vi "HW3_2017_BEEP.vi"() -> ()   [LabVIEW 2017]
panel:
  in  "OK Button 2":bool
  in  "Path":path
  in  "min":dbl
  in  "hour":dbl
  in  "OK Button":bool
  out "Boolean":bool
  in  "SET ALARM":bool
  out "ALARMING TIME":string
  out "DATE":string
  in  "reinstate":bool
  in  "sec":dbl
  in  "min":dbl
  in  "hour":dbl
  in  "reset":bool
  out "sec":dbl(knob) scale=0.0..60.0
  out "min":dbl(knob) scale=0.0..60.0
  out "hour":dbl(knob) scale=0.0..12.0
  in  "stop":bool
  out "new picture":picture
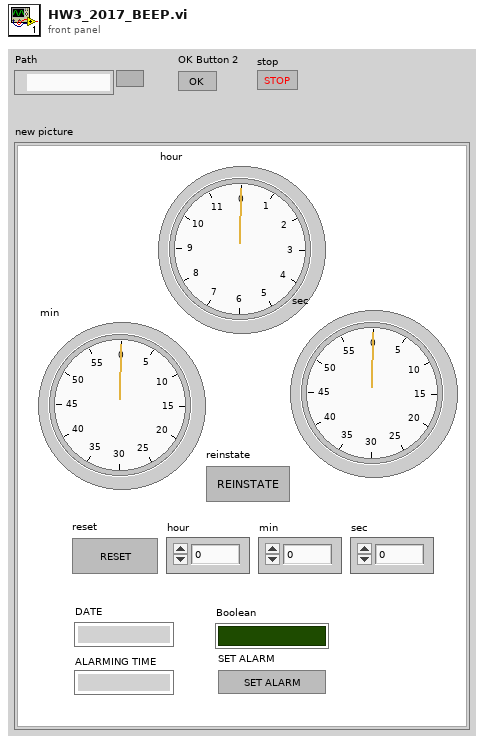
[diagram p1: front panel]
types:
  T1 = typedef "LVDateTimeRec.ctl" = cluster{"fractional second":dbl, "second":i32, "minute":i32, "hour":i32, "day of month":i32, "month":i32, "year":i32, "day of week":i32, "day of year":i32, "DST":i32}
  T2 = typedef "imagedata.ctl" = cluster{"image type":i32, "image depth":i32, "image":u8[], "mask":u8[], "colors":u32[], "Rectangle":cluster{"left":i16, "top":i16, "right":i16, "bottom":i16}}
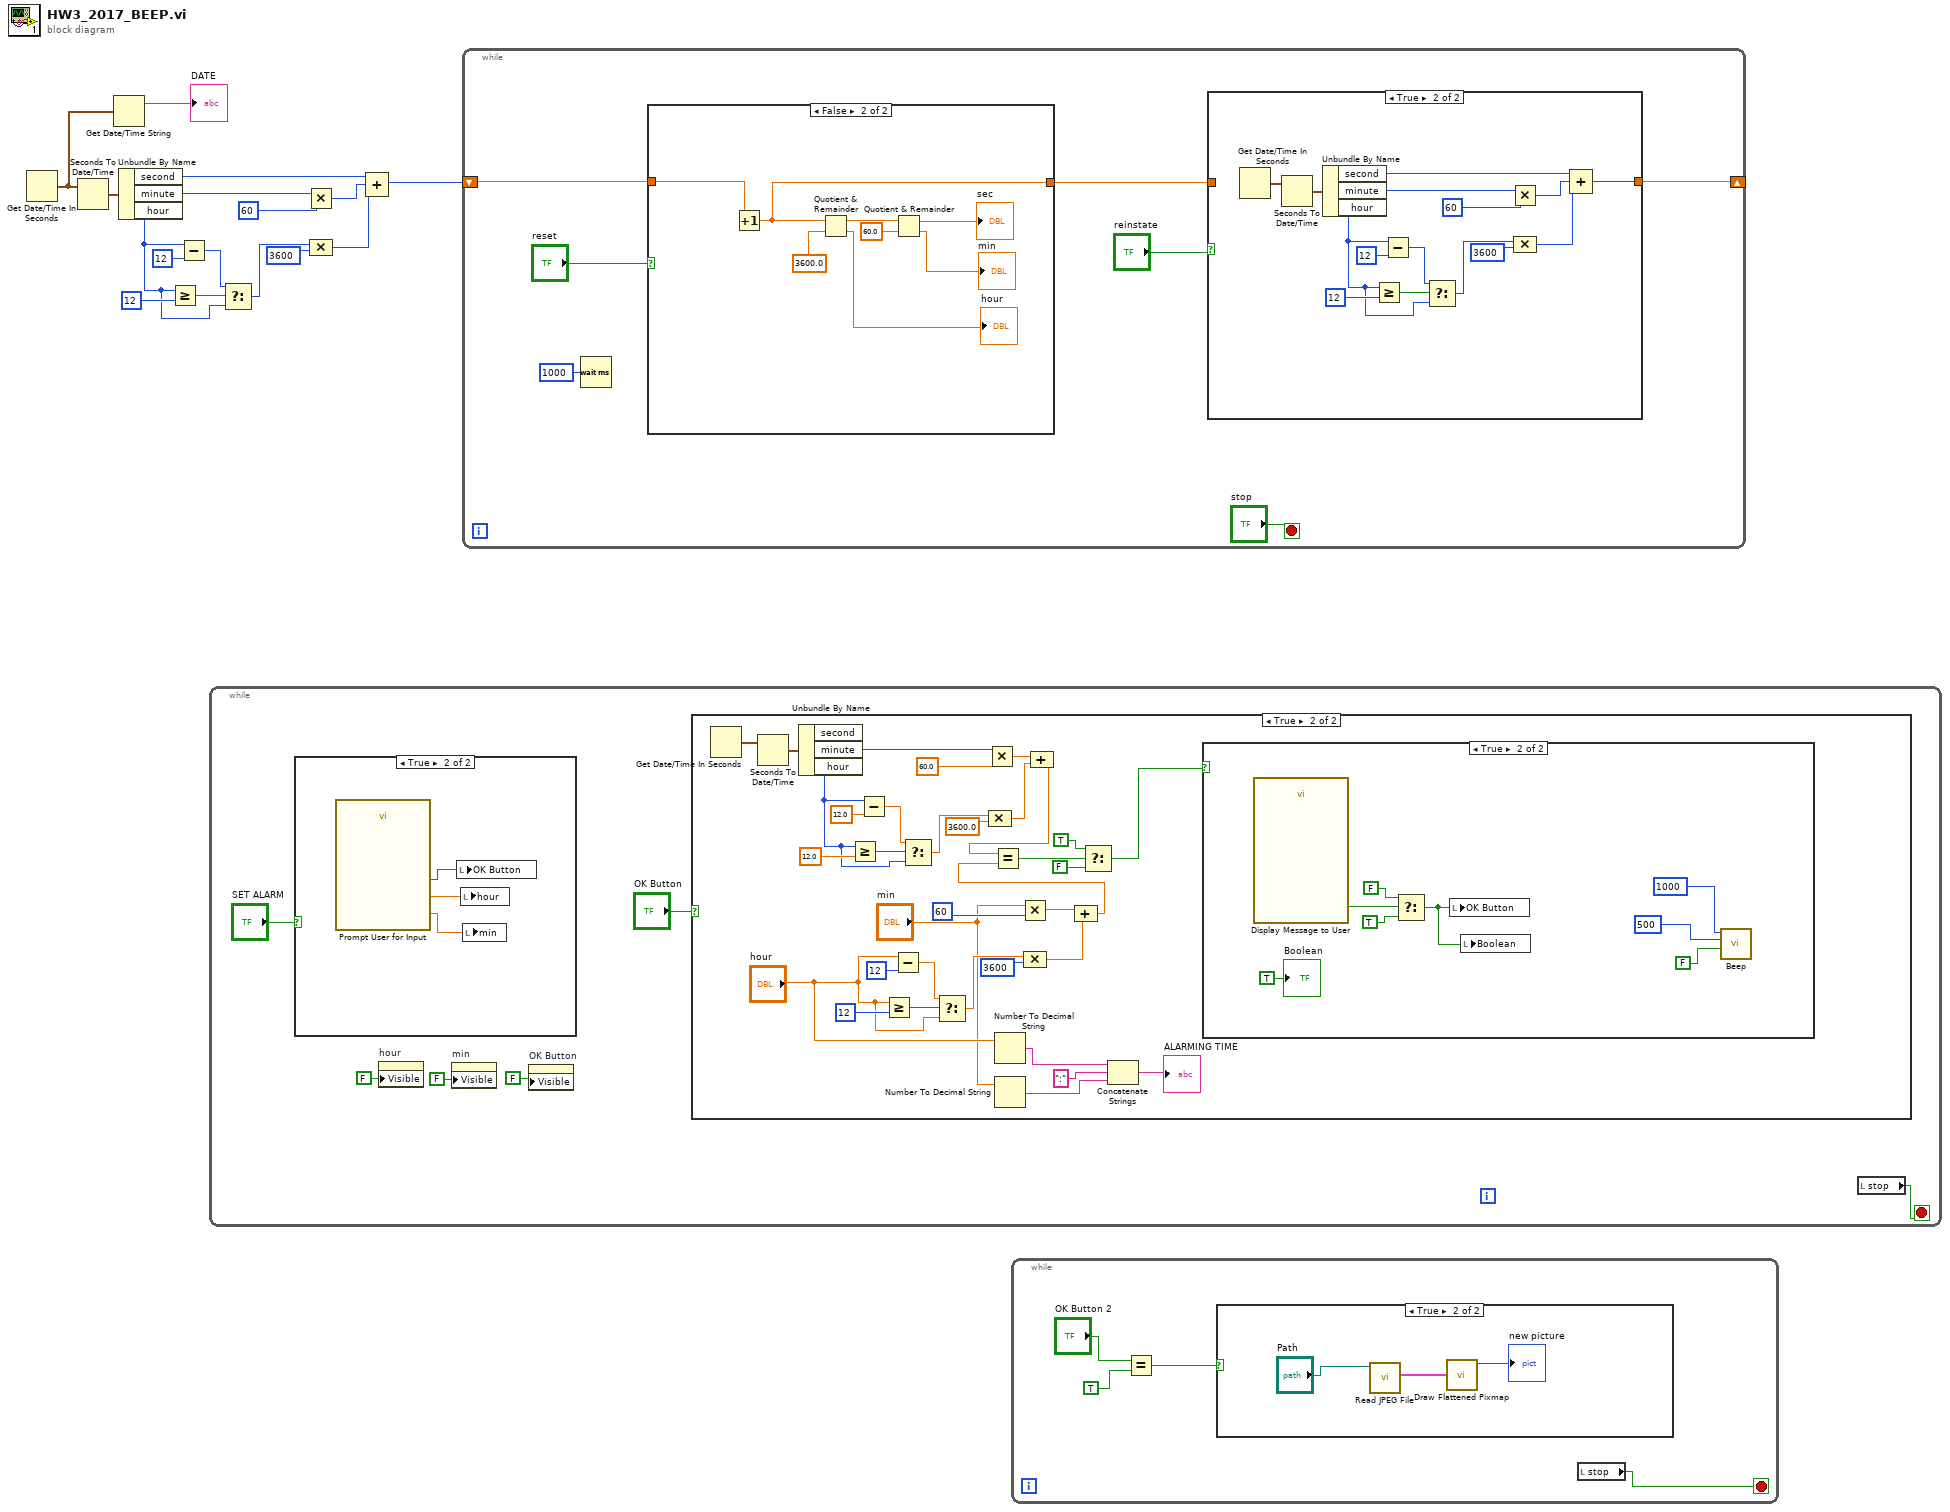
[diagram p0: block diagram]
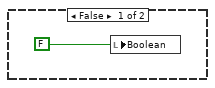
[diagram p4: hidden frame]
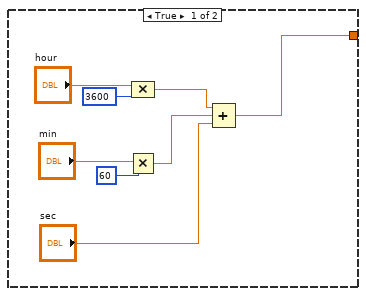
[diagram p7: hidden frame]
diagram:
  n1 = Get Date/Time In Seconds() -> (seconds since 1Jan1904=w5:timestamp)
  n2 = Seconds To Date/Time(time stamp (now)=w5) -> (date time rec=w14:T1)  [unwired: 1 in]
  n3 = Get Date/Time String(seconds (now)=w5) -> (date string=→"DATE":string)  [unwired: 2 in, 1 out]
  n4 = Unbundle By Name(w14) -> ("second"=w12:i32, "minute"=w13:i32, "hour"=w7:i32)
  n5 = Greater Or Equal?(x=w7, y=12) -> (x >= y?=w10:bool)
  n6 = Subtract(x=w7, y=12) -> (x-y=w8:i32)
  n7 = while {
    stop <- w18 stop-if-true
    n8 = case shown="True" "SET ALARM" {
      frame False {
      }
      frame True {
        n9 = call "Prompt User for Input"() -> ("Minute"=w68:dbl, "Hour"=w67:dbl, "OK"=w66:bool)  [unwired: 16 in, 1 out]
        n10 = local write "OK Button"(w66) -> ()
        n11 = local write "hour"(w67) -> ()
        n12 = local write "min"(w68) -> ()
      }
    }
    n13 = property on="hour" class="DigNum (strict)"("Visible"=FALSE) -> ()  [unwired: 2 in, 2 out]
    n14 = property on="min" class="DigNum (strict)"("Visible"=FALSE) -> ()  [unwired: 2 in, 2 out]
    n15 = property on="OK Button" class="Bool (strict)"("Visible"=FALSE) -> ()  [unwired: 2 in, 2 out]
    n16 = case shown="True" "OK Button" {
      frame False {
      }
      frame True {
        n17 = Get Date/Time In Seconds() -> (seconds since 1Jan1904=w26:timestamp)
        n18 = Seconds To Date/Time(time stamp (now)=w26) -> (date time rec=w29:T1)  [unwired: 1 in]
        n19 = Unbundle By Name(w29) -> ("minute"=w30:i32, "hour"=w23:i32)  [unwired: 1 out]
        n20 = Greater Or Equal?(x=w23, y=12.0) -> (x >= y?=w32:bool)
        n21 = Subtract(x=w23, y=12.0) -> (x-y=w34:dbl)
        n22 = Greater Or Equal?(x="hour", y=12) -> (x >= y?=w51:bool)
        n23 = Subtract(x="hour", y=12) -> (x-y=w49:dbl)
        n24 = Select(t=w34, s=w32, f=w23) -> (s? t:f=w35:dbl)
        n25 = Select(t=w49, s=w51, f="hour") -> (s? t:f=w48:dbl)
        n26 = Multiply(x=w30, y=60.0) -> (x*y=w36:dbl)
        n27 = Compound Arithmetic op=MULTIPLY(w35, 3600.0) -> (w37:dbl)
        n28 = Number To Decimal String(number="hour") -> (decimal integer string=w43:string)  [unwired: 1 in]
        n29 = Number To Decimal String(number="min") -> (decimal integer string=w41:string)  [unwired: 1 in]
        n30 = Multiply(x="min", y=60) -> (x*y=w54:dbl)
        n31 = Compound Arithmetic op=MULTIPLY(w48, 3600) -> (w53:dbl)
        n32 = Compound Arithmetic op=ADD(w36, w37) -> (w25:dbl)
        n33 = Compound Arithmetic op=ADD(w54, w53) -> (w47:dbl)
        n34 = Equal?(x=w25, y=w47) -> (x = y?=w46:bool)
        n35 = Select(t=TRUE, s=w46, f=FALSE) -> (s? t:f=w24:bool)
        n36 = Concatenate Strings(w43, ":", w41) -> (→"ALARMING TIME":string)
        n37 = case shown="True" w24 {
          frame False {
            n38 = local write "Boolean"(FALSE ("Boolean")) -> ()
          }
          frame True {
            n39 = call "Display Message to User"() -> ("OK"=w61:bool)  [unwired: 10 in, 1 out]
            n40 = Select(t=FALSE ("Boolean"), s=w61, f=TRUE) -> (s? t:f=w62:bool)
            n41 = local write "OK Button"(w62) -> ()
            n42 = local write "Boolean"(w62) -> ()
            n43 = call <vilib>:"Beep.vi"("use system alert? (T)"=FALSE ("Boolean"), "duration (msec)"=u32 500, "frequency (Hz)"=u32 1000) -> ()  [unwired: 9 in]
            "Boolean" <- TRUE ("Boolean")
          }
        }
      }
    }
    n44 = local read "stop"() -> (w18:bool)
  }
  n45 = Select(t=w8, s=w10, f=w7) -> (s? t:f=w6:i32)
  n46 = Multiply(x=w13, y=60) -> (x*y=w2:i32)
  n47 = Compound Arithmetic op=MULTIPLY(w6, 3600) -> (w1:i32)
  n48 = Compound Arithmetic op=ADD(w12, w2, w1) -> (w4:i32)
  n49 = while {
    shift-right: [w70] -> _
    shift-left: w4 -> [w74]
    stop <- "stop" stop-if-true
    n50 = Wait (ms)(milliseconds to wait=u32 1000) -> ()  [unwired: 1 out]
    n51 = case shown="False" "reset" {
      tunnel: w74 -> [_ w107]
      tunnel: [w92 w100] -> w71
      frame True {
        n52 = Multiply(x="min", y=60) -> (x*y=w94:dbl)
        n53 = Compound Arithmetic op=MULTIPLY("hour", 3600) -> (w95:dbl)
        n54 = Compound Arithmetic op=ADD(w95, w94, "sec") -> (w92:dbl)
      }
      frame False {
        n55 = Increment(x=w107) -> (x+1=w100:dbl)
        n56 = Quotient & Remainder(x=w100, y=3600.0) -> (x-y*floor(x/y)=w105:dbl, floor(x/y)=→"hour":dbl)
        n57 = Quotient & Remainder(x=w105, y=60.0) -> (x-y*floor(x/y)=→"sec":dbl, floor(x/y)=→"min":dbl)
      }
    }
    n58 = case shown="True" "reinstate" {
      tunnel: w71 -> [w76 _]
      tunnel: [w76 w77] -> w70
      frame False {
      }
      frame True {
        n59 = Get Date/Time In Seconds() -> (seconds since 1Jan1904=w88:timestamp)
        n60 = Seconds To Date/Time(time stamp (now)=w88) -> (date time rec=w87:T1)  [unwired: 1 in]
        n61 = Unbundle By Name(w87) -> ("second"=w84:i32, "minute"=w86:i32, "hour"=w79:i32)
        n62 = Greater Or Equal?(x=w79, y=12) -> (x >= y?=w82:bool)
        n63 = Subtract(x=w79, y=12) -> (x-y=w80:i32)
        n64 = Select(t=w80, s=w82, f=w79) -> (s? t:f=w78:i32)
        n65 = Multiply(x=w86, y=60) -> (x*y=w89:i32)
        n66 = Compound Arithmetic op=MULTIPLY(w78, 3600) -> (w85:i32)
        n67 = Compound Arithmetic op=ADD(w84, w89, w85) -> (w77:i32)
      }
    }
  }
  n68 = while {
    stop <- w108 stop-if-true
    n69 = Equal?(x="OK Button 2", y=TRUE) -> (x = y?=w109:bool)
    n70 = case shown="True" w109 {
      frame False {
      }
      frame True {
        n71 = call <vilib>:"Read JPEG File.vi"("path to JPEG file"="Path") -> ("image data"=w113:T2)  [unwired: 8 in, 2 out]
        n72 = call <vilib>:"Draw Flattened Pixmap.vi"("image data"=w113) -> ("new picture"=→"new picture":picture)  [unwired: 8 in]
      }
    }
    n73 = local read "stop"() -> (w108:bool)
  }
